vi "发送close TCP Client.vi"(7 "Message Priority (Normal)":T1=enum."Normal" caption="消息优先级（标准）", 8 "error in (no error)":errorcluster caption="错误输入（无错误）", 11 "Message Enqueuer":refnum<class "Message Enqueuer.lvclass"> caption="消息待入队列") -> (0 "error out":errorcluster caption="错误输出", 3 "Message Enqueuer out":refnum<class "Message Enqueuer.lvclass"> caption="消息待入队列输出")   [LabVIEW 2022 SP3, in "LS-H600-TCP Client.lvlib" / "close TCP Client消息.lvclass"]
doc: "本VI将消息发送至操作者。"
uses:
  <vilib>/ActorFramework/Message Enqueuer/Message Enqueuer.lvclass
  <vilib>/ActorFramework/Message Enqueuer/Message Priority.ctl
  C:/Program Files (x86)/National Instruments/LabVIEW 2022/vi.lib/ActorFramework/Message/Message.lvclass
  <vilib>/ActorFramework/Message Enqueuer/Message Enqueuer.lvclass/Message Enqueuer.ctl
  <vilib>/ActorFramework/Message Priority Queue/Priority Enqueue.vi
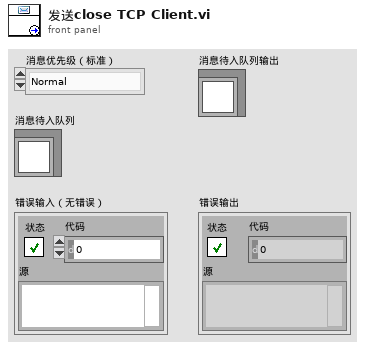
[diagram p1: front panel]
types:
  T1 = typedef "Actor Framework.lvlib/Message Enqueuer.lvclass/Message Priority.ctl" = enum16{"Low", "Normal", "High"}
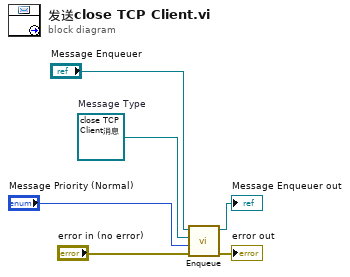
[diagram p0: block diagram]
diagram:
  w3 = refnum<class "close TCP Client消息.lvclass"> refnum  # Message Type
  n1 = call <vilib>:"Enqueue.vi"("error in (no error)"="error in (no error)", "Message Priority (Normal)"="Message Priority (Normal)", "Message"=w3, "Message Enqueuer in"="Message Enqueuer") -> ("error out"=→"error out":errorcluster, "Message Enqueuer out"=→"Message Enqueuer out":refnum<class "Message Enqueuer.lvclass">)  [unwired: 6 in]
